vi "Handle Core Error.vi"(8 "error in (no error)":errorcluster, 11 "Response Core in":refnum<class "Response Core.lvclass">) -> (0 "error out":errorcluster, 3 "Response Core out":refnum<class "Response Core.lvclass">)   [LabVIEW 2020, in "Publisher.lvlib" / "Response Core.lvclass"]
doc: "Handle Response Core errors at the end of the Response Msg Send method.\n\nThe default implementation does nothing."
uses:
  Response Core.lvclass
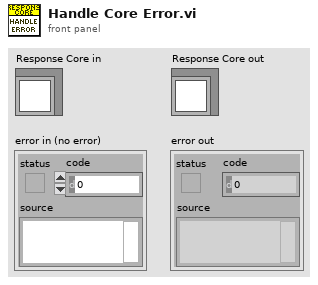
[diagram p1: front panel]
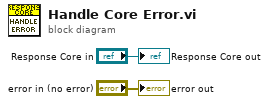
[diagram p0: block diagram]
diagram:
  "error out" <- "error in (no error)"
  "Response Core out" <- "Response Core in"
